vi "TDT-Write Tag.vi"(0 "RPcox":refnum<k7>, 5 "Name":string, 7 "Value":sgl, 11 "error in":errorcluster) -> (4 "RPcox Out":refnum<k7>, 15 "error out":errorcluster)   [LabVIEW 2020]
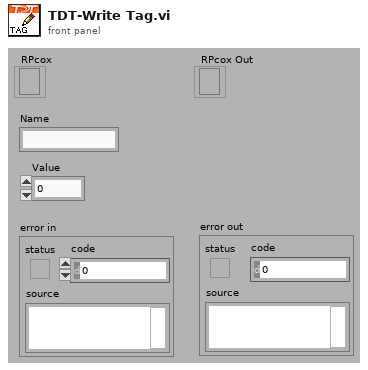
[diagram p1: front panel]
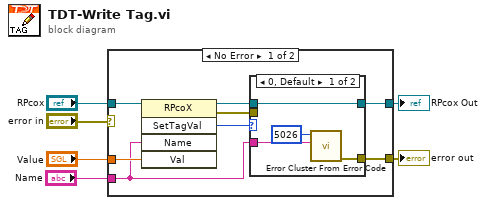
[diagram p0: block diagram]
diagram:
  n1 = case shown="No Error" "error in" {
    selector: "error in" -> [_ w22]
    tunnel: "Value" -> [w14 _]
    tunnel: "RPcox" -> [w11 w21]
    tunnel: [w9 w22] -> w4
    tunnel: [w8 w21] -> w3
    tunnel: "Name" -> [w7 _]
    frame No Error {
      n2 = invoke class="RPcoX" method="SetTagVal"(reference=w11, "Name"=w7, "Val"=w14) -> (reference out=w12:refnum<k7>, error out=w10:errorcluster, "SetTagVal"=w13:i32)  [unwired: 2 in, 2 out]
      n3 = case shown="0, Default" w13 {
        tunnel: w7 -> [w17 _]
        tunnel: w12 -> [w18 w20]
        tunnel: w10 -> [_ w19]
        tunnel: [w18 w20] -> w8
        tunnel: [w15 w19] -> w9
        frame 0, Default {
          n4 = call <vilib>:"Error Cluster From Error Code.vi"("error message (\"\")"=w17, "error code (0)"=5026) -> ("error out"=w15:errorcluster)  [unwired: 7 in]
        }
        frame 1 {
        }
      }
    }
    frame Error {
    }
  }
  "error out" <- w4
  "RPcox Out" <- w3
